vi "MultiChannelfFeedbackCooling (FPGA)_PIDXYZ_LockIn.vi"() -> ()   [LabVIEW 2016]
doc: "This VI will read single point values from 4 channels of a R Series board at a specified rate."
uses:
  <vilib>/rvi/Emulation/niFpgaGetClockAttributes.vi
  <vilib>/rvi/Emulation/niFpgaSctlEmulationGetInTimedLoop.vi
  <vilib>/rvi/Emulation/niFpgaEmulationReportErrorSimple.vi
  <vilib>/rvi/eio/common/nirviEmuTemplateMethod_errors.vi
  <vilib>/rvi/Memory/Memory_Emulation/nirvimemoryFastEmulation.vi
  <vilib>/rvi/Memory/Memory_Emulation/nirvimemoryEmulation.vi
  <vilib>/rvi/Emulation/niFpgaEmulationIsFPGAContextNoSignature.vi
  <vilib>/rvi/DataTransferAndStorage/Container/Common/niFpgaContainerGetUniqueNameForEmu.vi
  <vilib>/rvi/Emulation/niFpgaProcessEmulError.vi
  <vilib>/rvi/errors/nirviReportUnexpectedCaseInternalError (U32).vi
  <vilib>/rvi/Memory/Memory_Emulation/niFpgaMemoryEmulationCacheClearOnFirstRun.vi
  <vilib>/rvi/Memory/Memory_Emulation/nirvimemoryEmulationManagerCache_MakeExclusive.vi
  <vilib>/rvi/Memory/Memory_Emulation/niFpgaMemoryEmulationValidateCache.vi
  <vilib>/rvi/Memory/Memory_Emulation/nirvimemoryEmulationManagerCache_InsertValue.vi
  <vilib>/Utility/error.llb/Clear Errors.vi
  <vilib>/rvi/Memory/Memory_Emulation/nirvimemoryEmulationManagerCache_ReleaseExclusive.vi
  <vilib>/rvi/Memory/Memory_Emulation/nirvimemoryEmulationManagerCache_GetValue.vi
  <vilib>/rvi/Memory/Memory_Emulation/nirvimemoryEmulationManagerCache_SetValue.vi
  <vilib>/rvi/Emulation/niFpgaSctlEmulationResourceMgr.vi
  <vilib>/rvi/Emulation/niFpgaCriticalErrorInLSC.vi
  <vilib>/eio/EIONode/EIONode.xnode
  <vilib>/rvi/DataTransferAndStorage/Container/XNode/niFpgaContainer.xnode
  <vilib>/rvi/FXPMathLib/FxpInterpret/XNode/nifxpmath_Interpret.xnode
panel:
  in  "final filter coeff X before":i32[](array[numeric])=[-955995012, 2025731616, 1001305, -1023351008, 2092954700, 1034533]
  in  "final filter coeff X":i32[](array[numeric])=[-955995012, 2025731616, 1001305, -1023351008, 2092954700, 1034533]
  in  "final filter coeff Y before":i32[](array[numeric])=[-955995012, 2025731616, 1001305, -1023351008, 2092954700, 1034533]
  in  "final filter coeff Y":i32[](array[numeric])=[-955995012, 2025731616, 1001305, -1023351008, 2092954700, 1034533]
  in  "final filter coeff Z":i32[](array[numeric])=[-955995012, 2025731616, 1001305, -1023351008, 2092954700, 1034533]
  in  "final filter coeff Z before":i32[](array[numeric])=[-955995012, 2025731616, 1001305, -1023351008, 2092954700, 1034533]
  in  "LP Coeff Z before":i32[](array[numeric])=[1008310688, 32715568]
  in  "LP Coeff Z":i32[](array[numeric])=[1008310688, 32715568]
  in  "LP Coeff X":i32[](array[numeric])=[1008310688, 32715568]
  in  "LP Coeff X before":i32[](array[numeric])=[1008310688, 32715568]
  in  "LP Coeff Y before":i32[](array[numeric])=[1008310688, 32715568]
  in  "LP Coeff Y":i32[](array[numeric])=[1008310688, 32715568]
  in  "Upper lim Z before":fxp<+/-,16,16>
  in  "Lower lim Z before":fxp<+/-,16,16>
  in  "Upper lim Y before":fxp<+/-,16,16>
  in  "Lower lim Y before":fxp<+/-,16,16>
  in  "Upper lim X before":fxp<+/-,16,16>
  in  "Lower lim X before":fxp<+/-,16,16>
  in  "HP coeff band X before":i32[](array[numeric])=[-850883994, 1909449570, 958518847, -975456236, 2033039520, 1020559395]
  in  "LP Coeff band X before":i32[](array[numeric])=[-955995012, 2025731616, 1001305, -1023351008, 2092954700, 1034533]
  in  "LP Coeff band X":i32[](array[numeric])=[-955995012, 2025731616, 1001305, -1023351008, 2092954700, 1034533]
  in  "HP Coeff band X":i32[](array[numeric])=[-850883994, 1909449570, 958518847, -975456236, 2033039520, 1020559395]
  in  "dg band X before":fxp<+/-,24,12>
  in  "dg band X":fxp<+/-,24,12>
  in  "HP Coeff X before":i32[](array[numeric])=[946630756, 1010186290]
  in  "HP Coeff X":i32[](array[numeric])=[946630756, 1010186290]
  in  "Use X PID before":bool
  out "AI X before chamber plot":i16
  in  "X before Setpoint":i16
  out "tot_fb X plot":i16
  out "fb X before chamber plot":i16
  in  "DC offset X":i16
  in  "pg X before":fxp<+/-,24,12>
  in  "ig X before":fxp<+/-,24,6>
  in  "dg X before":fxp<+/-,24,12>
  out "fb X plot":i16
  in  "ig X":fxp<+/-,24,6>
  in  "Lower lim X":fxp<+/-,16,16>
  in  "Upper lim X":fxp<+/-,16,16>
  in  "dg X":fxp<+/-,24,12>
  in  "pg X":fxp<+/-,24,12>
  out "AI X plot":i16
  in  "X Setpoint":i16
  in  "HP coeff band Y before":i32[](array[numeric])=[-850883994, 1909449570, 958518847, -975456236, 2033039520, 1020559395]
  in  "LP Coeff band Y before":i32[](array[numeric])=[-955995012, 2025731616, 1001305, -1023351008, 2092954700, 1034533]
  in  "LP Coeff band Y":i32[](array[numeric])=[-955995012, 2025731616, 1001305, -1023351008, 2092954700, 1034533]
  in  "HP Coeff band Y":i32[](array[numeric])=[-850883994, 1909449570, 958518847, -975456236, 2033039520, 1020559395]
  in  "dg band Y before":fxp<+/-,24,12>
  in  "dg band Y":fxp<+/-,24,12>
  in  "HP Coeff Y before":i32[](array[numeric])=[946630756, 1010186290]
  in  "HP Coeff Y":i32[](array[numeric])=[946630756, 1010186290]
  in  "Use Y PID before":bool
  out "AI Y before chamber plot":i16
  in  "Y before Setpoint":i16
  out "tot_fb Y plot":i16
  out "fb Y before chamber plot":i16
  in  "DC offset Y":i16
  in  "pg Y before":fxp<+/-,24,12>
  in  "ig Y before":fxp<+/-,24,6>
  in  "dg Y before":fxp<+/-,24,12>
  out "fb Y plot":i16
  in  "ig Y":fxp<+/-,24,6>
  in  "Lower lim Y":fxp<+/-,16,16>
  in  "Upper lim Y":fxp<+/-,16,16>
  in  "dg Y":fxp<+/-,24,12>
  in  "pg Y":fxp<+/-,24,12>
  out "AI Y plot":i16
  in  "Y Setpoint":i16
  in  "EOM_offset":i16
  in  "EOM_seed":u32=4294967295 caption="seed"
  in  "EOM reset":bool caption="reset"
  in  "EOM_threshold":i16
  in  "EOM_amplitude":i16
  in  "HP coeff band Z before":i32[](array[numeric])=[-850883994, 1909449570, 958518847, -975456236, 2033039520, 1020559395]
  in  "LP Coeff band Z before":i32[](array[numeric])=[-955995012, 2025731616, 1001305, -1023351008, 2092954700, 1034533]
  in  "LP Coeff band Z":i32[](array[numeric])=[-955995012, 2025731616, 1001305, -1023351008, 2092954700, 1034533]
  in  "HP Coeff band Z":i32[](array[numeric])=[-850883994, 1909449570, 958518847, -975456236, 2033039520, 1020559395]
  in  "dg band Z before":fxp<+/-,24,12>
  in  "dg band Z":fxp<+/-,24,12>
  in  "data_buffer3":i16
  in  "Arb gain (ch2)":fxp<+/-,24,12>=0.5 caption="RMS"
  in  "HP Coeff Z before":i32[](array[numeric])=[946630756, 1010186290]
  in  "HP Coeff Z":i32[](array[numeric])=[946630756, 1010186290]
  in  "Use Z PID before":bool
  out "AI Z before chamber plot":i16
  in  "Z before Setpoint":i16
  out "tot_fb Z plot":i16
  out "fb Z before chamber plot":i16
  in  "DC offset Z":i16
  in  "pg Z before":fxp<+/-,24,12>
  in  "ig Z before":fxp<+/-,24,6>
  in  "dg Z before":fxp<+/-,24,12>
  out "fb Z plot":i16
  in  "ig Z":fxp<+/-,24,6>
  out "written_address":u32
  in  "ready_to_write":bool
  in  "Arb steps per cycle":u16
  in  "data_buffer2":i16
  in  "data_buffer_1":i16
  in  "write_address":u16
  in  "Arb gain (ch1)":fxp<+/-,24,12>=0.5 caption="RMS"
  in  "Arb gain (ch0)":fxp<+/-,24,12>=0.5 caption="RMS"
  in  "Lower lim Z":fxp<+/-,16,16>
  in  "Upper lim Z":fxp<+/-,16,16>
  in  "dg Z":fxp<+/-,24,12>
  in  "pg Z":fxp<+/-,24,12>
  out "AI Z plot":i16
  in  "Z Setpoint":i16
  in  "Count(uSec)":u32
  out "FPGA Error Out":errorcluster
  in  "Stop":bool
  # "test"
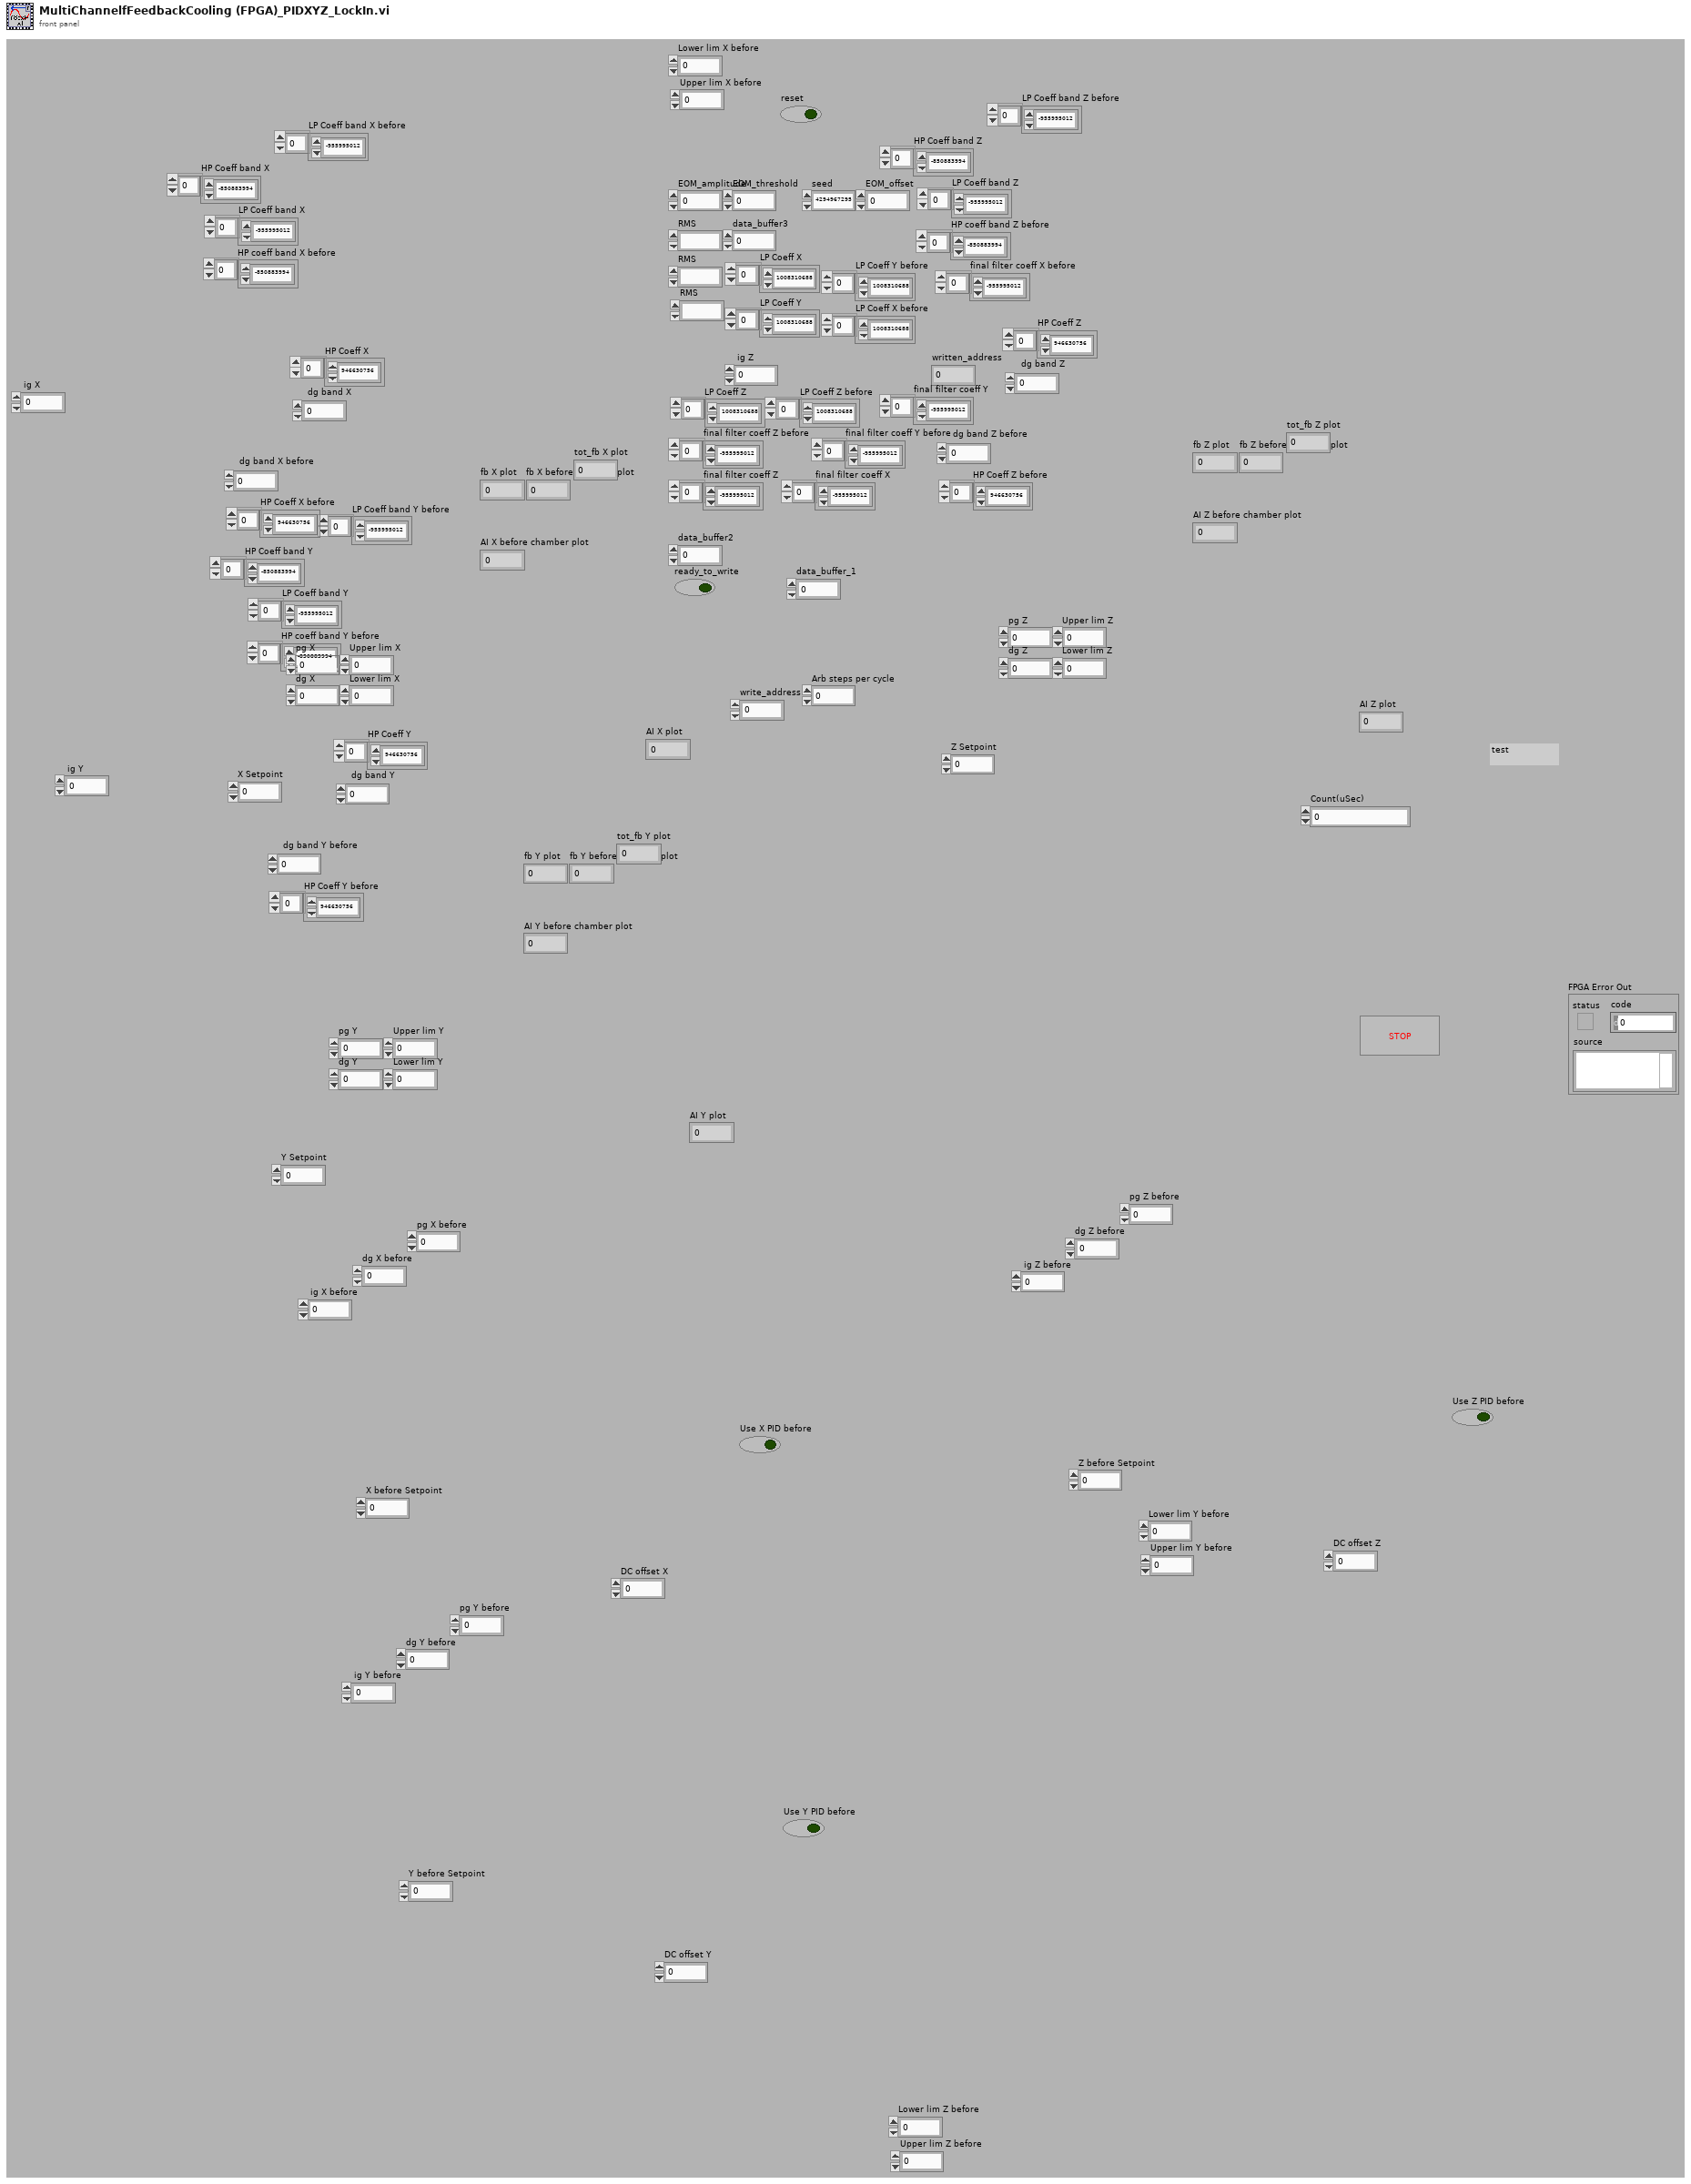
[diagram p1: front panel]
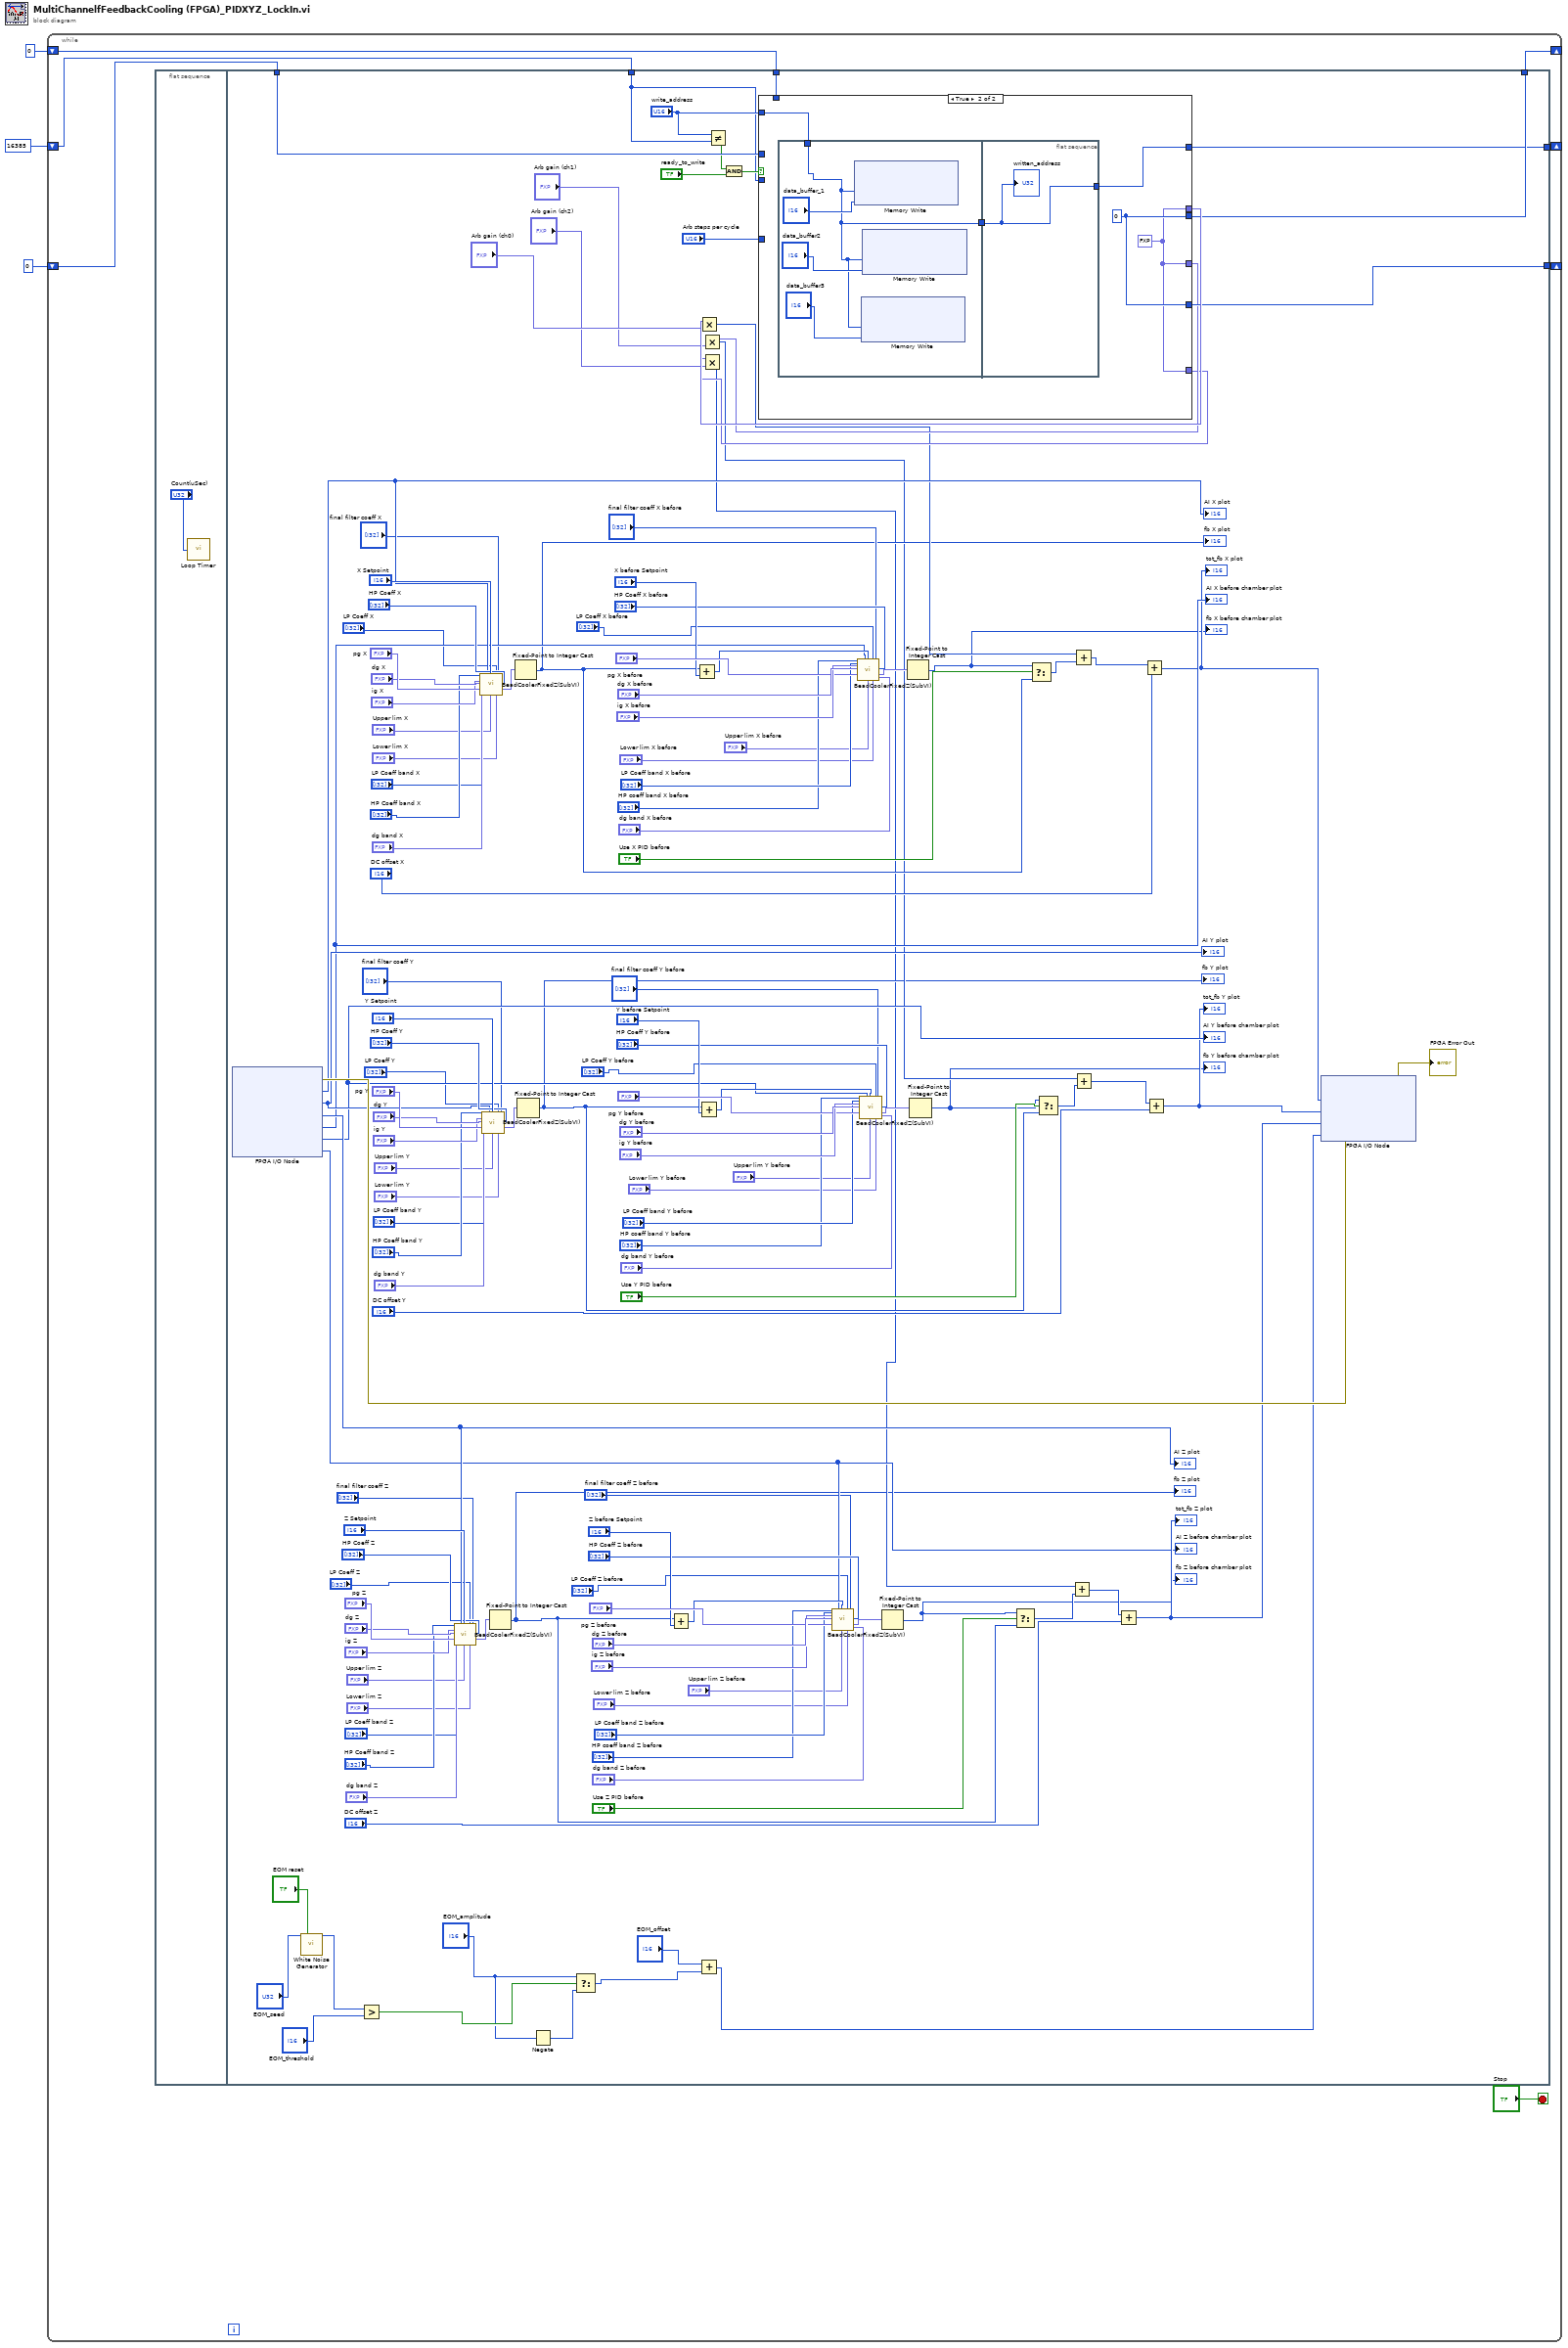
[diagram p0: block diagram]
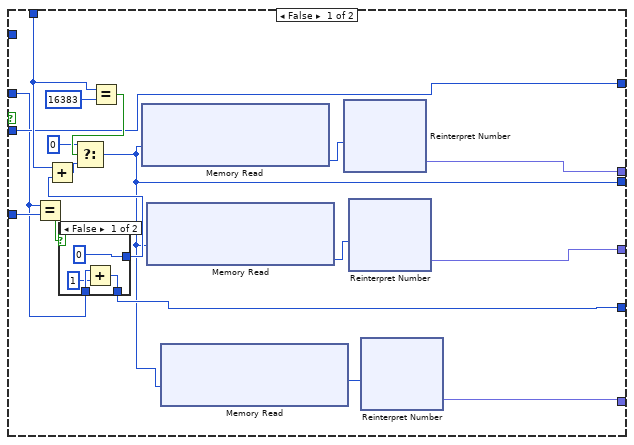
[diagram p2: hidden frame]
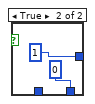
[diagram p3: hidden frame]
diagram:
  n1 = while {
    shift-right: [w9] -> _
    shift-left: u16 0 ("t") -> [w8]
    shift-right: [w7] -> _
    shift-left: u16 0 ("t") -> [w4]
    shift-right: [w6] -> _
    shift-left: u32 16385 ("write_address") -> [w5]
    stop <- "Stop" stop-if-true
    n2 = flat-sequence {
      tunnel: [w144] -> w9
      tunnel: w8 -> [w143]
      tunnel: [w141] -> w7
      tunnel: w4 -> [w140]
      tunnel: [w139] -> w6
      tunnel: w5 -> [w132]
      frame #0 {
        n3 = call "Loop Timer"("Count(uSec)"="Count(uSec)") -> ()  [unwired: 1 out]
      }
      frame #1 {
        n4 = xnode "FPGA I/O Node"() -> ("error out"=w151:errorcluster, "Connector0/AI0"=w47:i16, "Connector0/AI1"=w74:i16, "Connector0/AI2"=w130:i16, "Connector0/AI3"=w46:i16, "Connector0/AI4"=w72:i16, "Connector0/AI5"=w73:i16)  [unwired: 7 in, 6 out]
        "AI Z plot" <- w130
        "AI Z before chamber plot" <- w73
        "AI Y plot" <- w74
        "AI Y before chamber plot" <- w72
        "AI X plot" <- w47
        "AI X before chamber plot" <- w46
        n5 = call "White Noise Generator"("seed"="EOM_seed", "reset"="EOM reset") -> ("white noise out"=w109:i16)  [unwired: 13 in]
        n6 = Greater?(x=w109, y="EOM_threshold") -> (0:w107:bool)
        n7 = call "BeadCoolerFixedZ(SubVI).vi"("hp coeff band"="HP Coeff band Z", "lp coeff band"="LP Coeff band Z", "ig"="ig Z", "dg"="dg Z", "pg"="pg Z", "dg band"="dg band Z", "AI0"=w130, "Dc Pos"="Z Setpoint", "Upper lim"="Upper lim Z", "lp coeff"="LP Coeff Z", "Lower lim"="Lower lim Z", "final filter coeff"="final filter coeff Z", "hp coeff"="HP Coeff Z") -> ("Output"=w119:fxp<+/-,16,16>)  [unwired: 14 in]
        n8 = call "BeadCoolerFixedZ(SubVI).vi"("hp coeff band"="HP Coeff band X", "lp coeff band"="LP Coeff band X", "ig"="ig X", "dg"="dg X", "pg"="pg X", "dg band"="dg band X", "AI0"=w47, "Dc Pos"="X Setpoint", "Upper lim"="Upper lim X", "lp coeff"="LP Coeff X", "Lower lim"="Lower lim X", "final filter coeff"="final filter coeff X", "hp coeff"="HP Coeff X") -> ("Output"=w57:fxp<+/-,16,16>)  [unwired: 14 in]
        n9 = call "BeadCoolerFixedZ(SubVI).vi"("hp coeff band"="HP Coeff band Y", "lp coeff band"="LP Coeff band Y", "ig"="ig Y", "dg"="dg Y", "pg"="pg Y", "dg band"="dg band Y", "AI0"=w74, "Dc Pos"="Y Setpoint", "Upper lim"="Upper lim Y", "lp coeff"="LP Coeff Y", "Lower lim"="Lower lim Y", "final filter coeff"="final filter coeff Y", "hp coeff"="HP Coeff Y") -> ("Output"=w84:fxp<+/-,16,16>)  [unwired: 14 in]
        n10 = Fixed-Point to Integer Cast(1:w119) -> (0:w21:i16)
        "fb Z plot" <- w21
        n11 = Fixed-Point to Integer Cast(1:w57) -> (0:w25:i16)
        "fb X plot" <- w25
        n12 = Fixed-Point to Integer Cast(1:w84) -> (0:w23:i16)
        "fb Y plot" <- w23
        n13 = Negate(x="EOM_amplitude") -> (-x=w105:i16)
        n14 = Select(t="EOM_amplitude", s=w107, f=w105) -> (s? t:f=w101:i16)
        n15 = Add(x=w21, y="Z before Setpoint") -> (x+y=w118:i16)
        n16 = Add(x=w25, y="X before Setpoint") -> (x+y=w56:i16)
        n17 = Add(x=w23, y="Y before Setpoint") -> (x+y=w83:i16)
        n18 = Add(x="EOM_offset", y=w101) -> (x+y=w102:i16)
        n19 = Not Equal?(x="write_address", y=w132) -> (x != y?=w136:bool)
        n20 = And(x=w136, y="ready_to_write") -> (x .and. y?=w137:bool)
        n21 = case shown="True" w137 {
          tunnel: [w168 w176] -> w146
          tunnel: [w153 w180] -> w144
          tunnel: w143 -> [w161 _]
          tunnel: [w162 w176] -> w134
          tunnel: "Arb steps per cycle" -> [w160 _]
          tunnel: [w155 w180] -> w141
          tunnel: w140 -> [w156 _]
          tunnel: [w159 w178] -> w139
          tunnel: w132 -> [w159 _]
          tunnel: "write_address" -> [_ w177]
          tunnel: [w152 w176] -> w116
          frame False {
            n22 = Equal?(x=w156, y=w160) -> (x = y?=w158:bool)
            n23 = case shown="False" w158 {
              tunnel: [u16 0 ("y") u16 1 ("y")] -> w157
              tunnel: w156 -> [w172 _]
              tunnel: [w170 u16 0] -> w155
              frame False {
                n24 = Add(x=w172, y=u16 1) -> (x+y=w170:u16)
              }
              frame True {
              }
            }
            n25 = Add(x=w161, y=w157) -> (x+y=w164:u16)
            n26 = Equal?(x=w161, y=u16 16383) -> (x = y?=w166:bool)
            n27 = Select(t=u16 0, s=w166, f=w164) -> (s? t:f=w153:u16)
            n28 = xnode ("Memory Read")("Address"=w153) -> ("Data"=w169:i16)  [unwired: 1 in, 1 out]
            n29 = xnode ("Memory Read")("Address"=w153) -> ("Data"=w163:i16)  [unwired: 1 in, 1 out]
            n30 = xnode ("Memory Read")("Address"=w153) -> ("Data"=w154:i16)  [unwired: 1 in, 1 out]
            n31 = xnode "Reinterpret Number"("x"=w169) -> ("y"=w168:fxp<+/-,16,16>)
            n32 = xnode "Reinterpret Number"("x"=w163) -> ("y"=w162:fxp<+/-,16,16>)
            n33 = xnode "Reinterpret Number"("x"=w154) -> ("y"=w152:fxp<+/-,16,16>)
          }
          frame True {
            w180 = u16 0
            w176 = fxp<+/-,16,16> 0.0 ("y")
            n34 = flat-sequence {
              tunnel: [w182] -> w179
              tunnel: w177 -> [w182]
              tunnel: w179 -> [w185]
              tunnel: [w185] -> w178
              frame #0 {
                n35 = xnode ("Memory Write")("Address"=w182, "Data"="data_buffer_1") -> ()  [unwired: 1 in, 1 out]
                n36 = xnode ("Memory Write")("Address"=w182, "Data"="data_buffer3") -> ()  [unwired: 1 in, 1 out]
                n37 = xnode ("Memory Write")("Address"=w182, "Data"="data_buffer2") -> ()  [unwired: 1 in, 1 out]
              }
              frame #1 {
                "written_address" <- w185
              }
            }
          }
        }
        n38 = Multiply(x=w146, y="Arb gain (ch0)") -> (x*y=w26:i16)
        n39 = Multiply(x=w134, y="Arb gain (ch1)") -> (x*y=w24:i16)
        n40 = Multiply(x=w116, y="Arb gain (ch2)") -> (x*y=w22:i16)
        n41 = call "BeadCoolerFixedZ(SubVI).vi"("hp coeff band"="HP coeff band Z before", "lp coeff band"="LP Coeff band Z before", "ig"="ig Z before", "dg"="dg Z before", "pg"="pg Z before", "dg band"="dg band Z before", "AI0"=w73, "Dc Pos"=w118, "Upper lim"="Upper lim Z before", "lp coeff"="LP Coeff Z before", "Lower lim"="Lower lim Z before", "final filter coeff"="final filter coeff Z before", "hp coeff"="HP Coeff Z before") -> ("Output"=w126:fxp<+/-,16,16>)  [unwired: 14 in]
        n42 = call "BeadCoolerFixedZ(SubVI).vi"("hp coeff band"="HP coeff band X before", "lp coeff band"="LP Coeff band X before", "ig"="ig X before", "dg"="dg X before", "pg"="pg X before", "dg band"="dg band X before", "AI0"=w46, "Dc Pos"=w56, "Upper lim"="Upper lim X before", "lp coeff"="LP Coeff X before", "Lower lim"="Lower lim X before", "final filter coeff"="final filter coeff X before", "hp coeff"="HP Coeff X before") -> ("Output"=w63:fxp<+/-,16,16>)  [unwired: 14 in]
        n43 = call "BeadCoolerFixedZ(SubVI).vi"("hp coeff band"="HP coeff band Y before", "lp coeff band"="LP Coeff band Y before", "ig"="ig Y before", "dg"="dg Y before", "pg"="pg Y before", "dg band"="dg band Y before", "AI0"=w72, "Dc Pos"=w83, "Upper lim"="Upper lim Y before", "lp coeff"="LP Coeff Y before", "Lower lim"="Lower lim Y before", "final filter coeff"="final filter coeff Y before", "hp coeff"="HP Coeff Y before") -> ("Output"=w90:fxp<+/-,16,16>)  [unwired: 14 in]
        n44 = Fixed-Point to Integer Cast(1:w126) -> (0:w12:i16)
        "fb Z before chamber plot" <- w12
        n45 = Fixed-Point to Integer Cast(1:w63) -> (0:w18:i16)
        "fb X before chamber plot" <- w18
        n46 = Fixed-Point to Integer Cast(1:w90) -> (0:w15:i16)
        "fb Y before chamber plot" <- w15
        n47 = Select(t=w12, s="Use Z PID before", f=w21) -> (s? t:f=w14:i16)
        n48 = Select(t=w18, s="Use X PID before", f=w25) -> (s? t:f=w20:i16)
        n49 = Select(t=w15, s="Use Y PID before", f=w23) -> (s? t:f=w17:i16)
        n50 = Add(x=w22, y=w14) -> (x+y=w13:i16)
        n51 = Add(x=w26, y=w20) -> (x+y=w19:i16)
        n52 = Add(x=w24, y=w17) -> (x+y=w16:i16)
        n53 = Add(x=w13, y="DC offset Z") -> (x+y=w122:i16)
        "tot_fb Z plot" <- w122
        n54 = Add(x=w19, y="DC offset X") -> (x+y=w45:i16)
        "tot_fb X plot" <- w45
        n55 = Add(x=w16, y="DC offset Y") -> (x+y=w71:i16)
        "tot_fb Y plot" <- w71
        n56 = xnode "FPGA I/O Node"("error in"=w151, "Connector0/AO0"=w45, "Connector0/AO1"=w71, "Connector0/AO2"=w122, "Connector0/AO3"=w102) -> ("error out"=→"FPGA Error Out":errorcluster)  [unwired: 4 in, 4 out]
      }
    }
  }
